vi "VI Tree.vi"   [LabVIEW 2010, in "Tektronix DPO MSO 2000 4000 Series.lvlib"]
doc: "This is the instrument driver for Tektronix DPO (2k, 3k, 4k), MSO (2k, 3k, 4k), and MDO. The VI Tree displays all the user-callable VIs of the instrument driver in an organized table."
uses:
  <instrlib>/Tektronix DPO MSO 2000 4000 Series/Tektronix DPO MSO 2000 4000 Series.lvlib
  <instrlib>/Tektronix DPO MSO 2000 4000 Series/Public/Data/Data_Low Level/Fetch Waveform (Waveform Data Type).vi
  <instrlib>/Tektronix DPO MSO 2000 4000 Series/Public/Data/Read (Single Waveform).vi
  <instrlib>/Tektronix DPO MSO 2000 4000 Series/Public/Configure/Configure Math (Dual).vi
  <instrlib>/Tektronix DPO MSO 2000 4000 Series/Public/Configure/Configure Trigger (USB).vi
  <instrlib>/Tektronix DPO MSO 2000 4000 Series/Public/Configure/Configure Bus Source (I2C).vi
panel:
  # "(c) 2006 - 2012. National Instruments Corporation. ALL RIGHTS RESERVED."
  # "SEE DIAGRAM\nFOR VI TREE."
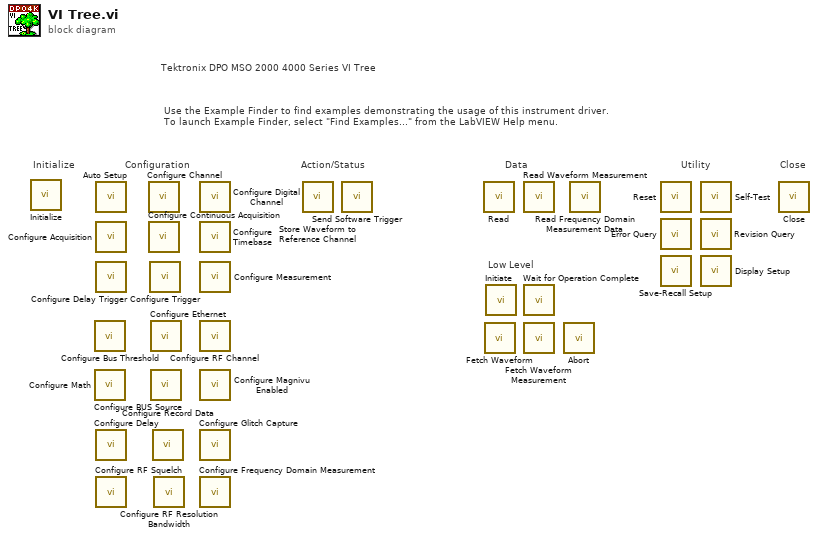
[diagram p0: block diagram]
diagram:
  # "Tektronix DPO MSO 2000 4000 Series VI Tree"
  # "Use the Example Finder to find examples demonstrating the usage of this instrument driver.\nTo launch Example Finder, select \"Find Examples...\" from the LabVIEW Help menu."
  # "Low Level"
  # "Action/Status"
  # "Configuration"
  # "Utility"
  # "Data"
  # "Close"
  # "Initialize"
  n1 = call <instrlib>:"Initialize.vi"() -> ()  [unwired: 10 in, 2 out]
  n2 = call <instrlib>:"Configure Bus Threshold.vi"() -> ()  [unwired: 10 in, 2 out]
  n3 = call-poly <instrlib>:"Configure Math.vi"() -> ()  [unwired: 10 in, 2 out]
  n4 = call <instrlib>:"Auto Setup.vi"() -> ()  [unwired: 10 in, 2 out]
  n5 = call <instrlib>:"Configure Acquisition.vi"() -> ()  [unwired: 10 in, 2 out]
  n6 = call <instrlib>:"Configure Delay Trigger.vi"() -> ()  [unwired: 14 in, 2 out]
  n7 = call <instrlib>:"Configure Delay.vi"() -> ()  [unwired: 10 in, 2 out]
  n8 = call <instrlib>:"Configure RF Squelch.vi"() -> ()  [unwired: 10 in, 2 out]
  n9 = call <instrlib>:"Configure Channel.vi"() -> ()  [unwired: 14 in, 2 out]
  n10 = call <instrlib>:"Configure Continuous Acquisition.vi"() -> ()  [unwired: 10 in, 2 out]
  n11 = call-poly <instrlib>:"Configure Trigger.vi"() -> ()  [unwired: 14 in, 2 out]
  n12 = call <instrlib>:"Configure Ethernet.vi"() -> ()  [unwired: 14 in, 2 out]
  n13 = call-poly <instrlib>:"Configure BUS Source.vi"() -> ()  [unwired: 14 in, 2 out]
  n14 = call <instrlib>:"Configure Record Data.vi"() -> ()  [unwired: 10 in, 2 out]
  n15 = call <instrlib>:"Configure RF Resolution Bandwidth.vi"() -> ()  [unwired: 14 in, 2 out]
  n16 = call <instrlib>:"Configure Digital Channel.vi"() -> ()  [unwired: 10 in, 2 out]
  n17 = call <instrlib>:"Configure Timebase.vi"() -> ()  [unwired: 10 in, 2 out]
  n18 = call <instrlib>:"Configure Measurement.vi"() -> ()  [unwired: 14 in, 2 out]
  n19 = call <instrlib>:"Configure RF Channel.vi"() -> ()  [unwired: 18 in, 2 out]
  n20 = call <instrlib>:"Configure Magnivu Enabled.vi"() -> ()  [unwired: 10 in, 2 out]
  n21 = call <instrlib>:"Configure Glitch Capture.vi"() -> ()  [unwired: 14 in, 2 out]
  n22 = call <instrlib>:"Configure Frequency Domain Measurement.vi"() -> ()  [unwired: 14 in, 2 out]
  n23 = call <instrlib>:"Store Waveform to Reference Channel.vi"() -> ()  [unwired: 10 in, 2 out]
  n24 = call <instrlib>:"Send Software Trigger.vi"() -> ()  [unwired: 10 in, 2 out]
  n25 = call-poly <instrlib>:"Read.vi"() -> ()  [unwired: 9 in, 3 out]
  n26 = call-poly <instrlib>:"Fetch Waveform.vi"() -> ()  [unwired: 9 in, 3 out]
  n27 = call <instrlib>:"Initiate.vi"() -> ()  [unwired: 10 in, 2 out]
  n28 = call <instrlib>:"Read Waveform Measurement.vi"() -> ()  [unwired: 9 in, 3 out]
  n29 = call <instrlib>:"Wait for Operation Complete.vi"() -> ()  [unwired: 10 in, 2 out]
  n30 = call <instrlib>:"Fetch Waveform Measurement.vi"() -> ()  [unwired: 9 in, 3 out]
  n31 = call <instrlib>:"Abort.vi"() -> ()  [unwired: 10 in, 2 out]
  n32 = call <instrlib>:"Read Frequency Domain Measurement Data.vi"() -> ()  [unwired: 7 in, 5 out]
  n33 = call <instrlib>:"Reset.vi"() -> ()  [unwired: 10 in, 2 out]
  n34 = call <instrlib>:"Error Query.vi"() -> ()  [unwired: 8 in, 4 out]
  n35 = call <instrlib>:"Save-Recall Setup.vi"() -> ()  [unwired: 10 in, 2 out]
  n36 = call <instrlib>:"Self-Test.vi"() -> ()  [unwired: 8 in, 4 out]
  n37 = call <instrlib>:"Revision Query.vi"() -> ()  [unwired: 8 in, 4 out]
  n38 = call <instrlib>:"Display Setup.vi"() -> ()  [unwired: 14 in, 2 out]
  n39 = call <instrlib>:"Close.vi"() -> ()  [unwired: 11 in, 1 out]
